vi "VI_principal K.vi"() -> ()   [LabVIEW 2025]
uses:
  <vilib>/LabVIEW Open Source Project/Epoch Date & Time/epoch.UNIX/Epoch.UNIX.lvclass
panel:
  out "Waveform Chart 2":waveform(dbl)(graph)
  out "Waveform Chart":waveform(dbl)(graph)
  out "output waveform 3":waveform(dbl)
  out "output waveform 2":waveform(dbl)
  in  "stop":bool
  out "Grafico fase A":waveform(dbl)(graph)
  out "output waveform":waveform(dbl)
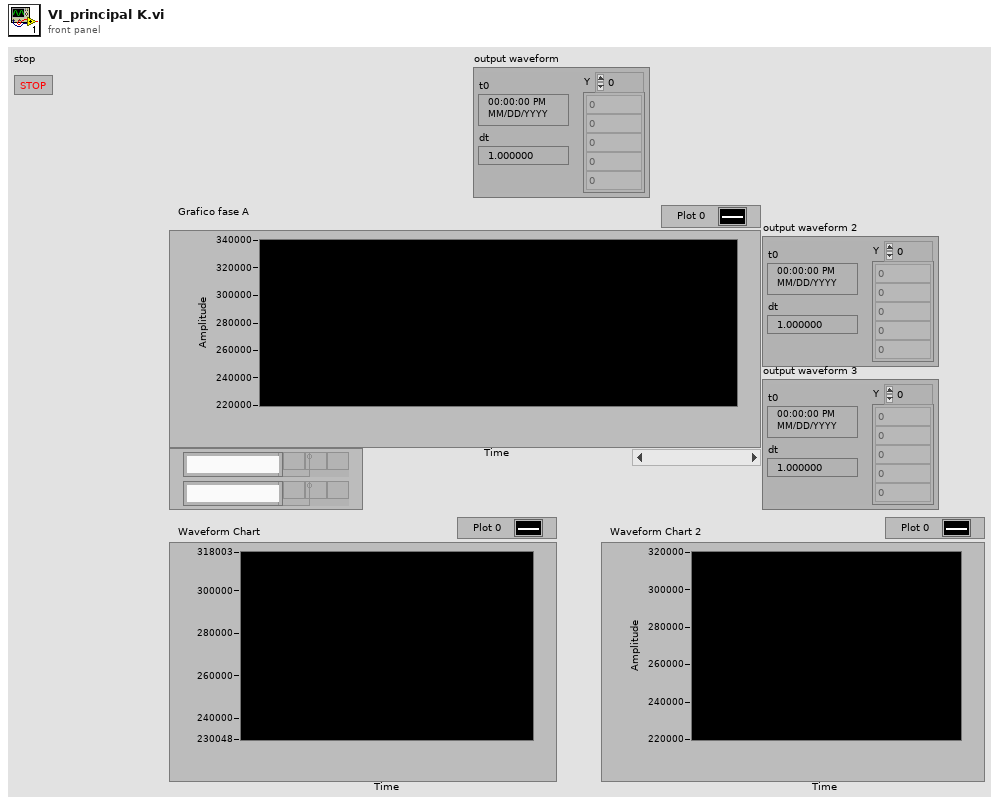
[diagram p1: front panel]
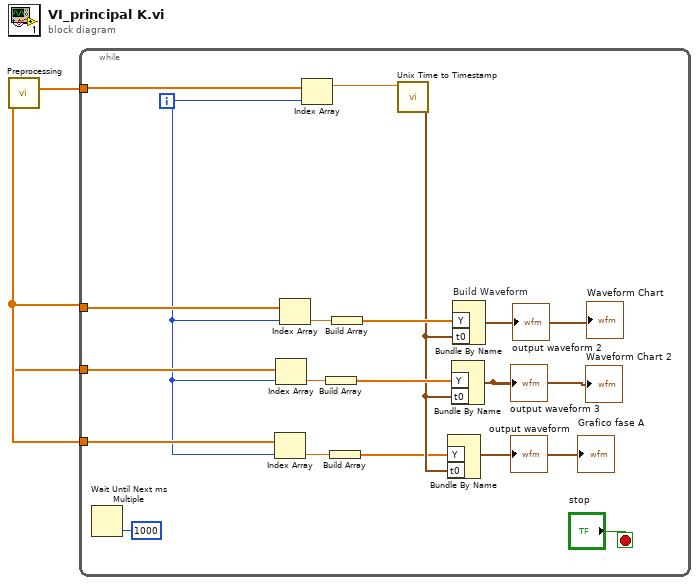
[diagram p0: block diagram]
diagram:
  n1 = call "Preprocessing.vi"() -> ("Timestamp"=w2:dbl[], "Potência instantänea A"=w3:dbl[], "Potência Ativa C"=w1:dbl[])  [unwired: 1 out]
  n2 = while {
    tunnel: w3 -> [w21]
    tunnel: w2 -> [w20]
    tunnel: w1 -> [w12]
    tunnel: w1 -> [w10]
    i -> [w9]
    stop <- "stop" stop-if-true
    n3 = Wait Until Next ms Multiple(millisecond multiple=u32 1000) -> ()  [unwired: 1 out]
    n4 = Index Array "Index Array"(array=w21, index=w9) -> (element=w18:dbl)
    n5 = Index Array "Index Array"(array=w12, index=w9) -> (element=w14:dbl)
    n6 = Index Array "Index Array"(array=w10, index=w9) -> (element=w11:dbl)
    n7 = Index Array "Index Array"(array=w20, index=w9) -> (element=w19:dbl)
    n8 = Build Array "Build Array"(w14) -> (w13:dbl[])
    n9 = Build Array "Build Array"(w18) -> (w6:dbl[])
    n10 = Build Array "Build Array"(w11) -> (w8:dbl[])
    n11 = call <vilib>:"Unix Time to Timestamp.vi"("Unix Time (s)"=w19) -> ("Timestamp"=w7:timestamp)  [unwired: 9 in, 1 out]
    n12 = Bundle By Name ("Build Waveform")("Y"=w6, "t0"=w7) -> (→"output waveform" →"Grafico fase A":waveform(dbl))  [unwired: 1 in]
    n13 = Bundle By Name ("Build Waveform")("Y"=w13, "t0"=w7) -> (→"output waveform 3" →"Waveform Chart 2":waveform(dbl))  [unwired: 1 in]
    n14 = Bundle By Name "Build Waveform"("Y"=w8, "t0"=w7) -> (→"output waveform 2" →"Waveform Chart":waveform(dbl))  [unwired: 1 in]
  }
